vi "Route CRD Data.vi"(8 "error in":errorcluster, 9 "ID":string, 10 "Data":refnum<class "Data.lvclass">, 11 "Controller in":refnum<class "Controller.lvclass">) -> (0 "error out":errorcluster, 3 "Controller out":refnum<class "Controller.lvclass">)   [LabVIEW 2014, in "Controller.lvlib" / "Controller.lvclass"]
doc: "Route the data from the devices for use by the CRD. This is updated when the data objects come in...."
uses:
  Controller.lvclass
  reusable/Data/Data.lvclass
  Controller.lvclass/Controller.ctl
  SuperActor/Ex Nested.lvclass/Ex Nested.ctl
  Devices/Alicat/Session Based/Data/Alicat Data.lvclass
  Devices/Alicat/Session Based/Data/Alicat Data.lvclass/Alicat Data.ctl
  Devices/Vaisala Probe/Data/Vaisala Data.lvclass
  Devices/Vaisala Probe/Data/Vaisala Data.lvclass/Vaisala Data.ctl
  Devices/PPT/Data/PPT Data.lvclass
  Devices/PPT/Data/PPT Data.lvclass/PPT Data.ctl
  SuperActor/Read Log Session.vi
  <userlib>/_Session Fwk/Session - Root.lvclass
  reusable/Session APIs/Session Log/System Log.lvclass
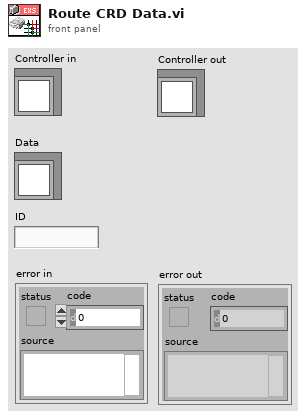
[diagram p1: front panel]
types:
  T1 = cluster{"P":sgl, "T":sgl, "Q":sgl, "Qsp":sgl, "Q0":sgl}
  T2 = typedef "Session - Root.lvclass/Session Handle.ctl" = refnum<data-value>
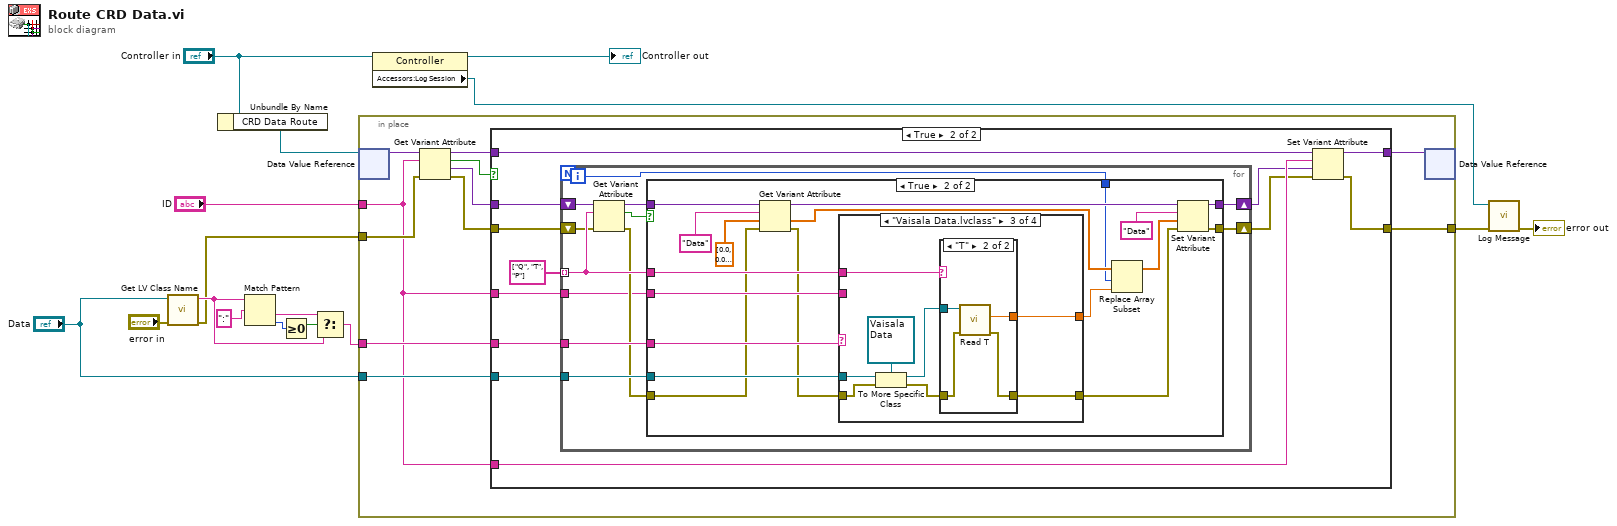
[diagram p0: block diagram]
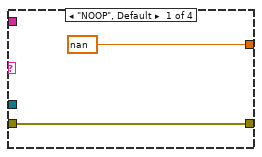
[diagram p4: hidden frame]
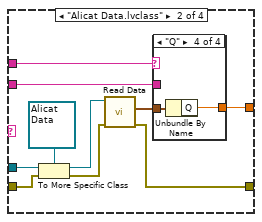
[diagram p5: hidden frame]
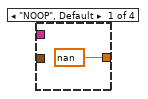
[diagram p6: hidden frame]
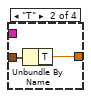
[diagram p7: hidden frame]
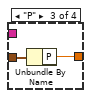
[diagram p8: hidden frame]
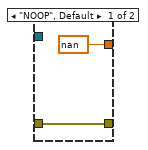
[diagram p9: hidden frame]
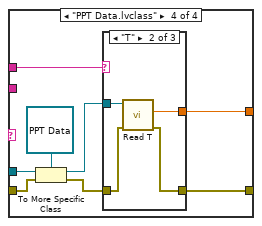
[diagram p10: hidden frame]
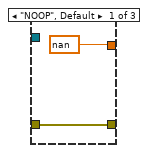
[diagram p11: hidden frame]
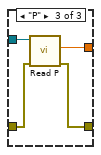
[diagram p12: hidden frame]
diagram:
  n1 = call <vilib>:"Get LV Class Name.vi"("error in (no error)"="error in", "object"="Data") -> ("error out"=w4:errorcluster, "class name"=w8:string)  [unwired: 8 in]
  n2 = Unbundle By Name("Controller in") -> ("CRD Data Route"=w6:refnum<data-value>)
  n3 = Match Pattern(string=w8, regular expression=":") -> (after substring=w9:string, offset past match=w11:i32)  [unwired: 1 in, 2 out]
  n4 = Greater Or Equal To 0?(x=w11) -> (x >= 0?=w10:bool)
  n5 = Select(t=w9, s=w10, f=w8) -> (s? t:f=w7:string)
  n6 = in-place {
    in-place-border: "ID" -> [w17]
    in-place-border: w7 -> [w22]
    in-place-border: "Data" -> [w21]
    in-place-border: w4 -> [w20]
    in-place-border: [w18] -> w14
    n7 = in-place-dvr #1(w6) -> (w27:variant)  [unwired: 1 out]
    n8 = Get Variant Attribute(Variant=w27, name=w17, error in=w20) -> (duplicate Variant=w25:variant, found=w26:bool, value=w23:variant, error out=w19:errorcluster)  [unwired: 1 in]
    n9 = case shown="True" w26 {
      tunnel: w25 -> [w29 w40]
      tunnel: [w29 w39] -> w24
      tunnel: w23 -> [_ w31]
      tunnel: w17 -> [_ w35]
      tunnel: w22 -> [_ w38]
      tunnel: w21 -> [_ w37]
      tunnel: w19 -> [w28 w30]
      tunnel: [w28 w36] -> w18
      tunnel: w17 -> [_ w34]
      frame False {
      }
      frame True {
        n10 = for {
          tunnel: string[] ["Q", "T", "P"] -> [w47] mode=indexing
          shift-right: [w50] -> w33
          shift-left: w31 -> [w53]
          tunnel: w38 -> [w49]
          tunnel: w37 -> [w48]
          shift-right: [w44] -> w32
          shift-left: w30 -> [w46]
          tunnel: w34 -> [w43]
          i -> [w42]
          n11 = Get Variant Attribute(Variant=w53, name=w47, error in=w46) -> (duplicate Variant=w51:variant, found=w52:bool, error out=w45:errorcluster)  [unwired: 1 in, 1 out]
          n12 = case shown="True" w52 {
            tunnel: w51 -> [w55 w63]
            tunnel: [w55 w70] -> w50
            tunnel: w49 -> [_ w73]
            tunnel: w48 -> [_ w72]
            tunnel: w47 -> [_ w69]
            tunnel: w45 -> [w54 w61]
            tunnel: [w54 w67] -> w44
            tunnel: w43 -> [_ w66]
            tunnel: w42 -> [_ w56]
            frame False {
            }
            frame True {
              n13 = Get Variant Attribute(Variant=w63, name="Data", default value (empty Variant)=dbl[] [0.0, 0.0, 0.0], error in=w61) -> (duplicate Variant=w62:variant, value=w58:dbl[], error out=w60:errorcluster)  [unwired: 1 out]
              n14 = case shown="\"Vaisala Data.lvclass\"" w73 {
                tunnel: w72 -> [_ w85 w100 w114]
                tunnel: [nan w81 w96 w111] -> w59
                tunnel: w69 -> [_ w80 w98 w110]
                tunnel: w60 -> [w74 w79 w95 w109]
                tunnel: [w74 w77 w93 w107] -> w68
                tunnel: w66 -> [_ w76 _ _]
                frame "NOOP", Default {
                }
                frame "Alicat Data.lvclass" {
                  n15 = To More Specific Class(target class=refnum<class "Alicat Data.lvclass"> refnum ("Alicat Lib.lvlib:Alicat Data"), reference=w85, error in=w79) -> (specific class reference=w83:refnum<class "Alicat Data.lvclass">, error out=w78:errorcluster)
                  n16 = call "Read Data.vi"("error in (no error)"=w78, "Alicat Data in"=w83) -> ("error out"=w77:errorcluster, "Data"=w82:T1)  [unwired: 7 in, 1 out]
                  n17 = case shown="\"Q\"" w80 {
                    tunnel: [nan w87 w89 w91] -> w81
                    tunnel: w82 -> [_ w88 w90 w92]
                    tunnel: w76 -> [_ _ _ _]
                    frame "NOOP", Default {
                    }
                    frame "T" {
                      n18 = Unbundle By Name(w88) -> ("T"=w87:sgl)
                    }
                    frame "P" {
                      n19 = Unbundle By Name(w90) -> ("P"=w89:sgl)
                    }
                    frame "Q" {
                      n20 = Unbundle By Name(w92) -> ("Q"=w91:sgl)
                    }
                  }
                }
                frame "Vaisala Data.lvclass" {
                  n21 = To More Specific Class(target class=refnum<class "Vaisala Data.lvclass"> refnum ("Vaisala Library.lvlib:Vaisala Data"), reference=w100, error in=w95) -> (specific class reference=w97:refnum<class "Vaisala Data.lvclass">, error out=w94:errorcluster)
                  n22 = case shown="\"T\"" w98 {
                    tunnel: w97 -> [_ w106]
                    tunnel: [nan w105] -> w96
                    tunnel: w94 -> [w101 w104]
                    tunnel: [w101 w103] -> w93
                    frame "NOOP", Default {
                    }
                    frame "T" {
                      n23 = call "Read T.vi"("error in (no error)"=w104, "Vaisala Data in"=w106) -> ("error out"=w103:errorcluster, "T"=w105:dbl)  [unwired: 7 in, 1 out]
                    }
                  }
                }
                frame "PPT Data.lvclass" {
                  n24 = To More Specific Class(target class=refnum<class "PPT Data.lvclass"> refnum ("PPT Library.lvlib:PPT Data"), reference=w114, error in=w109) -> (specific class reference=w112:refnum<class "PPT Data.lvclass">, error out=w108:errorcluster)
                  n25 = case shown="\"T\"" w110 {
                    tunnel: w112 -> [_ w120 w124]
                    tunnel: [nan w119 w123] -> w111
                    tunnel: w108 -> [w115 w118 w122]
                    tunnel: [w115 w117 w121] -> w107
                    frame "NOOP", Default {
                    }
                    frame "T" {
                      n26 = call "Read T.vi"("error in (no error)"=w118, "PPT Data in"=w120) -> ("error out"=w117:errorcluster, "T"=w119:dbl)  [unwired: 7 in, 1 out]
                    }
                    frame "P" {
                      n27 = call "Read P.vi"("error in (no error)"=w122, "PPT Data in"=w124) -> ("error out"=w121:errorcluster, "P"=w123:dbl)  [unwired: 7 in, 1 out]
                    }
                  }
                }
              }
              n28 = Replace Array Subset(array=w58, new element=w59, index=w56) -> (w57:dbl[])
              n29 = Set Variant Attribute(Variant=w62, name="Data", value=w57, error in=w68) -> (Variant out=w70:variant, error out=w67:errorcluster)  [unwired: 1 out]
            }
          }
        }
        n30 = Set Variant Attribute(Variant=w40, name=w35, value=w33, error in=w32) -> (Variant out=w39:variant, error out=w36:errorcluster)  [unwired: 1 out]
      }
    }
    n31 = in-place-dvr #1(w24) -> ()  [unwired: 2 out]
  }
  n32 = property class="Controller"(reference="Controller in") -> (reference out=→"Controller out":refnum<class "Controller.lvclass">, "Accessors:Log Session"=w2:T2)  [unwired: 1 in, 1 out]
  n33 = call "Log Message.vi"("error in"=w14, "session in"=w2) -> ("error out"=→"error out":errorcluster)  [unwired: 8 in, 1 out]
